vi "Test Gantry Dispenser.vi"() -> ()   [LabVIEW 2011]
uses:
  Gantry Class.lvclass
panel:
  out "error out":errorcluster
  in  "Enable":bool
  in  "stop":bool
  in  "Config Folder":path=path "C:/Users/Husker/Desktop/gantry/Config"
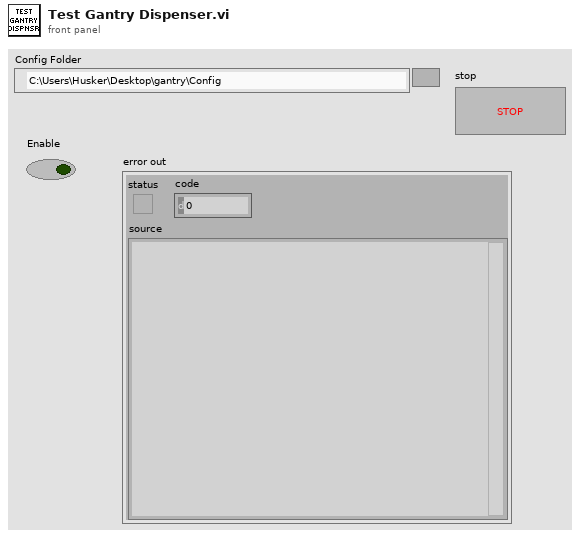
[diagram p1: front panel]
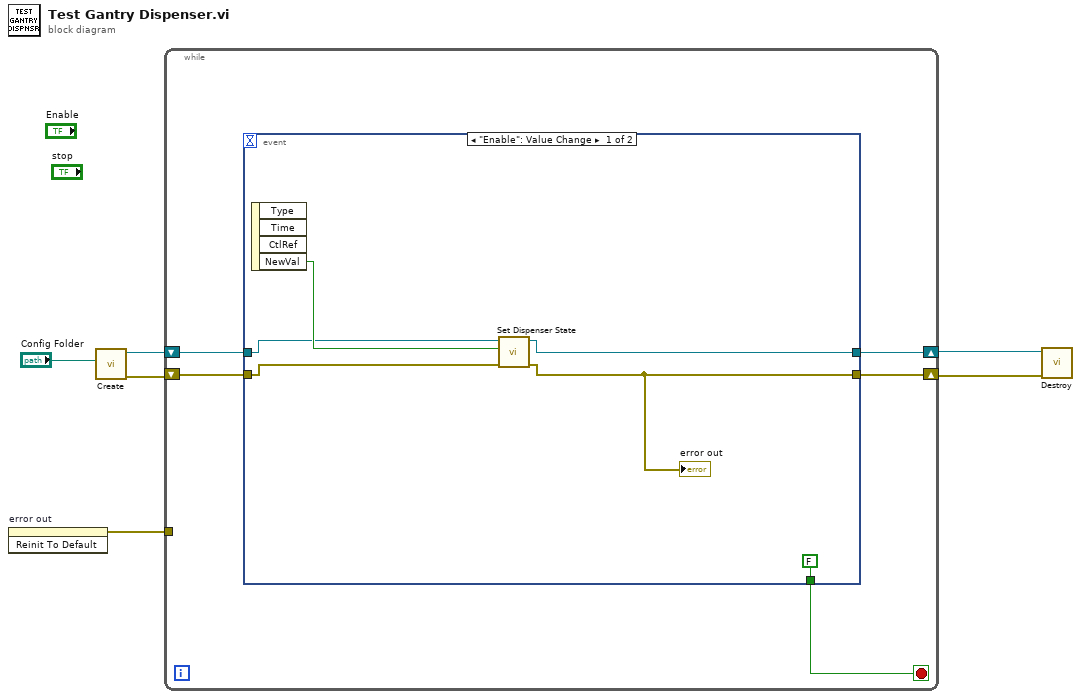
[diagram p0: block diagram]
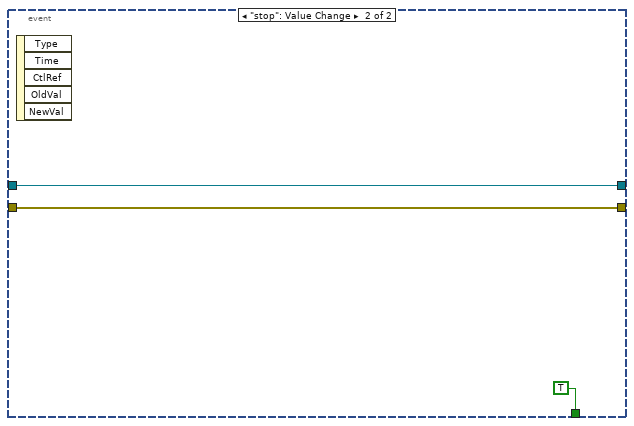
[diagram p2: hidden frame]
diagram:
  n1 = invoke on="error out" class="Clust (strict)" method="Reinit To Default"() -> (error out=w1:errorcluster)  [unwired: 3 in, 2 out]
  n2 = call "Create.vi"("Config Folder"="Config Folder") -> ("error out"=w4:errorcluster, "Gantry out"=w5:refnum<class "Gantry Class.lvclass">)  [unwired: 9 in]
  n3 = while {
    shift-right: [w10] -> w3
    shift-left: w5 -> [w11]
    shift-right: [w7] -> w2
    shift-left: w4 -> [w8]
    tunnel: w1 -> [_]
    stop <- w9 stop-if-true
    n4 = event shown="[0] \"Enable\": Value Change" {
      selector: _ -> [_ _]
      dyn-events: _ -> [_ _]
      timeout: _ -> [_ _]
      tunnel: w11 -> [w16 w19]
      tunnel: [w14 w19] -> w10
      tunnel: [FALSE TRUE] -> w9
      tunnel: w8 -> [w15 w18]
      tunnel: [w12 w18] -> w7
      event "Enable": Value Change {
        n5 = event-data() -> ("NewVal"=w17:bool)  [unwired: 1 in, 3 out]
        n6 = call-dynamic "Set Dispenser State.vi"("error in (no error)"=w15, "On/Off"=w17, "Gantry Class in"=w16) -> ("error out"=w12:errorcluster, "Gantry Class out"=w14:refnum<class "Gantry Class.lvclass">)  [unwired: 7 in]
        "error out" <- w12
      }
      event "stop": Value Change {
        n7 = event-data() -> ()  [unwired: 1 in, 5 out]
      }
    }
  }
  n8 = call "Destroy.vi"("error in"=w2, "Gantry Class in"=w3) -> ()  [unwired: 9 in, 1 out]
